vi "Init ConvBox.vi"(4 "system controller (T)":bool=TRUE, 6 "Assert Ren with IFC":bool, 7 "IST bit sense (T)":bool=TRUE, 8 "error in (no error)":errorcluster, 10 "Address":string, 11 "Serial Port":refnum<visa-resource-name>="Com1") -> (0 "error out":errorcluster, 3 "Serial Port Out":refnum<visa-resource-name>)   [LabVIEW 2019]
uses:
  <vilib>/Instr/_visa.llb/VISA Flush IO Buffer Mask.ctl
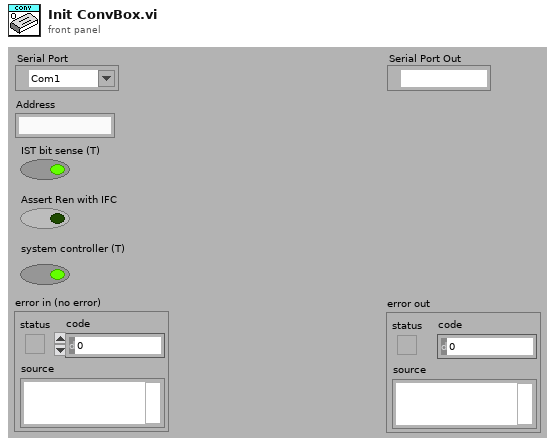
[diagram p1: front panel]
types:
  T1 = typedef "VISA Flush IO Buffer Mask.ctl" = u16
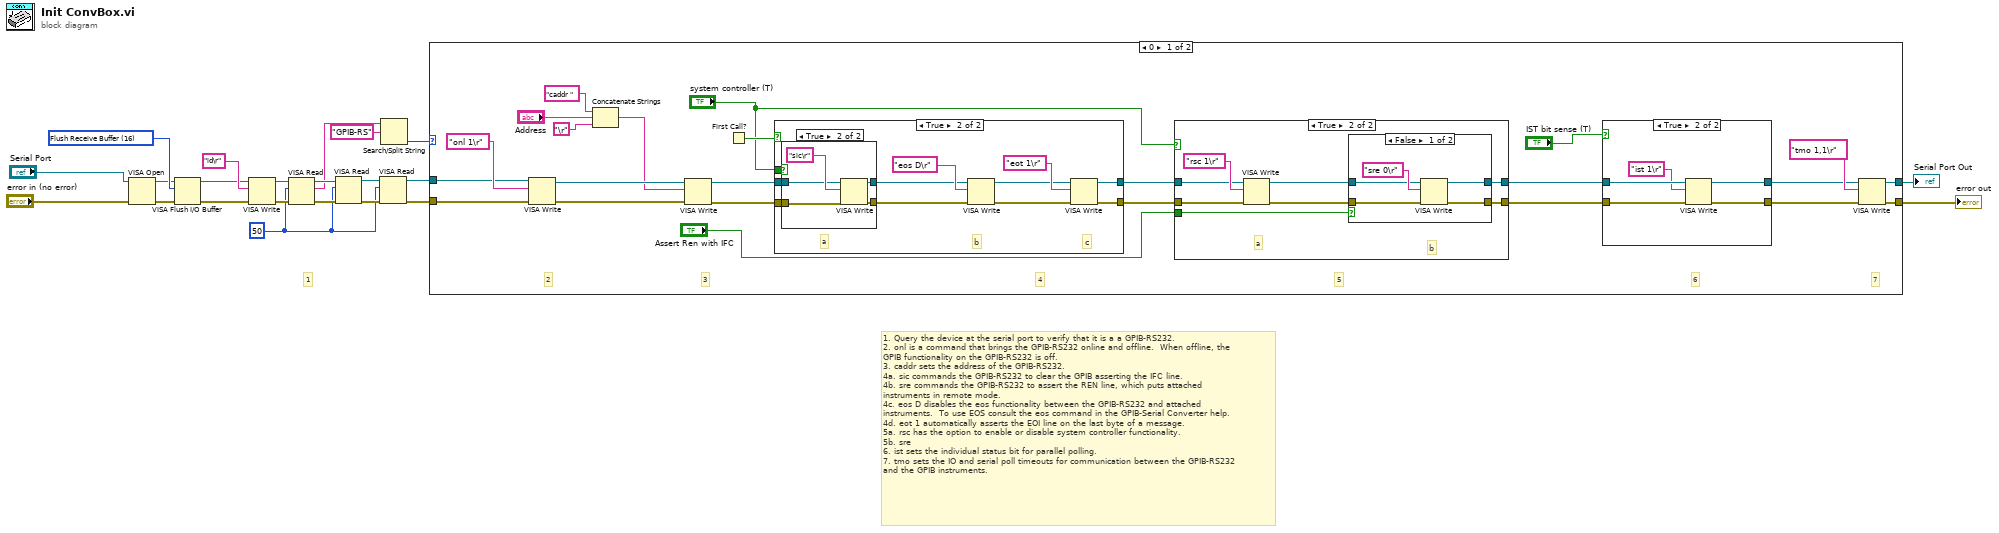
[diagram p0: block diagram]
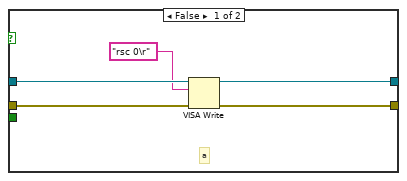
[diagram p3: hidden frame]
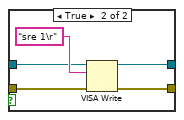
[diagram p4: hidden frame]
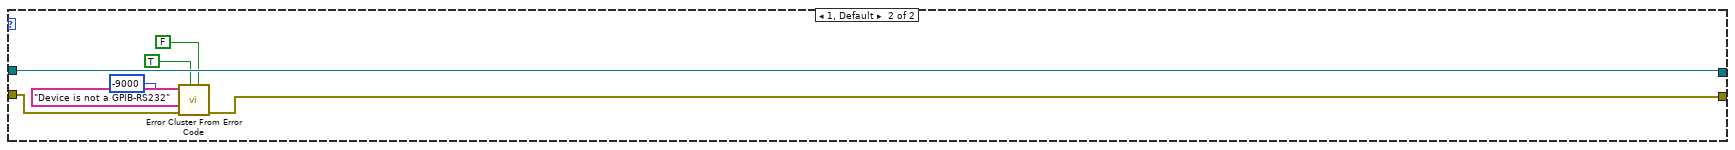
[diagram p7: hidden frame]
diagram:
  w8 = T1 16 items=["Flush Receive Buffer"=16, "Write Transmit Buffer to Device"=32, "Flush Receive Buffer (No I/O)"=64, "Flush Transmit Buffer"=128] ("Mask")
  w3 = u32 50 ("byte count")
  # "1. Query the device at the serial port to verify that it is a a GPIB-RS232.\n2. onl is a command that brings the GPIB-RS232 online and offline.  When offline, the\nGPIB functionality on the GPIB-RS232 is off.\n3. caddr sets the address of the GPIB-RS232.\n4a. sic commands the GPIB-RS232 to clear the GPIB asserting the IFC line.\n4b. sre commands the GPIB-RS232 to assert the REN line, which puts attached \ninstruments in remote mode.\n4c. eos D disables the eos functionality between the GPIB-RS232 and attached \ninstruments.  To use EOS consult the eos command in the GPIB-Serial Converter help.\n4d. eot 1 automatically asserts the EOI line on the last byte of a message.\n5a. rsc has the option to enable or disable system controller functionality.\n5b. sre\n6. ist sets the individual status bit for parallel polling.\n7. tmo sets the IO and serial poll timeouts for communication between the GPIB-RS232\nand the GPIB instruments."
  # "1"
  n1 = VISA Open(error in (no error)="error in (no error)", VISA resource name="Serial Port") -> (VISA resource name=w1:refnum<visa-resource-name>, error out=w2:errorcluster)  [unwired: 3 in]
  n2 = VISA Flush I/O Buffer(VISA resource name=w1, mask (16)=w8, error in (no error)=w2) -> (VISA resource name out=w7:refnum<visa-resource-name>, error out=w6:errorcluster)
  n3 = VISA Write(VISA resource name=w7, write buffer="id\r", error in (no error)=w6) -> (VISA resource name out=w17:refnum<visa-resource-name>, error out=w16:errorcluster)  [unwired: 1 out]
  n4 = VISA Read(VISA resource name=w17, byte count=w3, error in (no error)=w16) -> (VISA resource name out=w14:refnum<visa-resource-name>, read buffer=w11:string, error out=w15:errorcluster)  [unwired: 1 out]
  n5 = VISA Read(VISA resource name=w14, byte count=w3, error in (no error)=w15) -> (VISA resource name out=w12:refnum<visa-resource-name>, error out=w13:errorcluster)  [unwired: 2 out]
  n6 = VISA Read(VISA resource name=w12, byte count=w3, error in (no error)=w13) -> (VISA resource name out=w4:refnum<visa-resource-name>, error out=w5:errorcluster)  [unwired: 2 out]
  n7 = Search/Split String(string=w11, search string/char (-)="GPIB-RS") -> (offset of match=w9:i32)  [unwired: 1 in, 2 out]
  n8 = case shown="0" w9 {
    tunnel: [w24 w103] -> w22
    tunnel: [w25 w97] -> w21
    tunnel: w5 -> [w31 w101]
    tunnel: w4 -> [w30 w103]
    frame 0 {
      # "7"
      # "6"
      # "5"
      # "4"
      # "3"
      # "2"
      n9 = VISA Write(VISA resource name=w30, write buffer="onl 1\r", error in (no error)=w31) -> (VISA resource name out=w36:refnum<visa-resource-name>, error out=w39:errorcluster)  [unwired: 1 out]
      n10 = Concatenate Strings("caddr " ("write buffer"), "Address", "\r") -> (w34:string)
      n11 = VISA Write(VISA resource name=w36, write buffer=w34, error in (no error)=w39) -> (VISA resource name out=w37:refnum<visa-resource-name>, error out=w38:errorcluster)  [unwired: 1 out]
      n12 = First Call?() -> (First Call?: T/F=w46:bool)
      n13 = case shown="True" w46 {
        tunnel: w37 -> [w78 w89]
        tunnel: w38 -> [w77 w88]
        tunnel: [w78 w83] -> w44
        tunnel: [w77 w82] -> w43
        tunnel: "system controller (T)" -> [_ w81]
        frame False {
        }
        frame True {
          # "c"
          # "b"
          # "a"
          n14 = case shown="True" w81 {
            tunnel: w89 -> [w91 w95]
            tunnel: [w91 w94] -> w79
            tunnel: [w90 w93] -> w80
            tunnel: w88 -> [w90 w92]
            frame False {
            }
            frame True {
              n15 = VISA Write(VISA resource name=w95, write buffer="sic\r", error in (no error)=w92) -> (VISA resource name out=w94:refnum<visa-resource-name>, error out=w93:errorcluster)  [unwired: 1 out]
            }
          }
          n16 = VISA Write(VISA resource name=w79, write buffer="eos D\r", error in (no error)=w80) -> (VISA resource name out=w85:refnum<visa-resource-name>, error out=w84:errorcluster)  [unwired: 1 out]
          n17 = VISA Write(VISA resource name=w85, write buffer="eot 1\r", error in (no error)=w84) -> (VISA resource name out=w83:refnum<visa-resource-name>, error out=w82:errorcluster)  [unwired: 1 out]
        }
      }
      n18 = case shown="True" "system controller (T)" {
        tunnel: "Assert Ren with IFC" -> [_ w66]
        tunnel: w44 -> [w58 w64]
        tunnel: w43 -> [w55 w63]
        tunnel: [w57 w60] -> w42
        tunnel: [w56 w59] -> w41
        frame False {
          # "a"
          n19 = VISA Write(VISA resource name=w58, write buffer="rsc 0\r", error in (no error)=w55) -> (VISA resource name out=w57:refnum<visa-resource-name>, error out=w56:errorcluster)  [unwired: 1 out]
        }
        frame True {
          # "b"
          # "a"
          n20 = VISA Write(VISA resource name=w64, write buffer="rsc 1\r", error in (no error)=w63) -> (VISA resource name out=w62:refnum<visa-resource-name>, error out=w61:errorcluster)  [unwired: 1 out]
          n21 = case shown="False" w66 {
            tunnel: w62 -> [w70 w75]
            tunnel: w61 -> [w69 w74]
            tunnel: [w68 w73] -> w60
            tunnel: [w67 w72] -> w59
            frame False {
              n22 = VISA Write(VISA resource name=w70, write buffer="sre 0\r", error in (no error)=w69) -> (VISA resource name out=w68:refnum<visa-resource-name>, error out=w67:errorcluster)  [unwired: 1 out]
            }
            frame True {
              n23 = VISA Write(VISA resource name=w75, write buffer="sre 1\r", error in (no error)=w74) -> (VISA resource name out=w73:refnum<visa-resource-name>, error out=w72:errorcluster)  [unwired: 1 out]
            }
          }
        }
      }
      n24 = case shown="True" "IST bit sense (T)" {
        tunnel: w42 -> [w48 w53]
        tunnel: w41 -> [w47 w52]
        tunnel: [w48 w50] -> w26
        tunnel: [w47 w49] -> w27
        frame False {
        }
        frame True {
          n25 = VISA Write(VISA resource name=w53, write buffer="ist 1\r", error in (no error)=w52) -> (VISA resource name out=w50:refnum<visa-resource-name>, error out=w49:errorcluster)  [unwired: 1 out]
        }
      }
      n26 = VISA Write(VISA resource name=w26, write buffer="tmo 1,1\r", error in (no error)=w27) -> (VISA resource name out=w24:refnum<visa-resource-name>, error out=w25:errorcluster)  [unwired: 1 out]
    }
    frame 1, Default {
      n27 = call <vilib>:"Error Cluster From Error Code.vi"("is warning? (False)"=FALSE, "show call chain? (False)"=TRUE, "error in (no error)"=w101, "error message (\"\")"="Device is not a GPIB-RS232" ("error message (\"\")"), "error code (0)"=-9000) -> ("error out"=w97:errorcluster)  [unwired: 4 in]
    }
  }
  "Serial Port Out" <- w22
  "error out" <- w21
